vi "Test.vi"() -> ()   [LabVIEW 2014]
uses:
  support/kinectRead [BodyFrame].vi
  <vilib>/vision/NI_Vision_Development_Module.lvlib
panel:
  out "Image":T1(plugin-control)
  in  "stop":bool
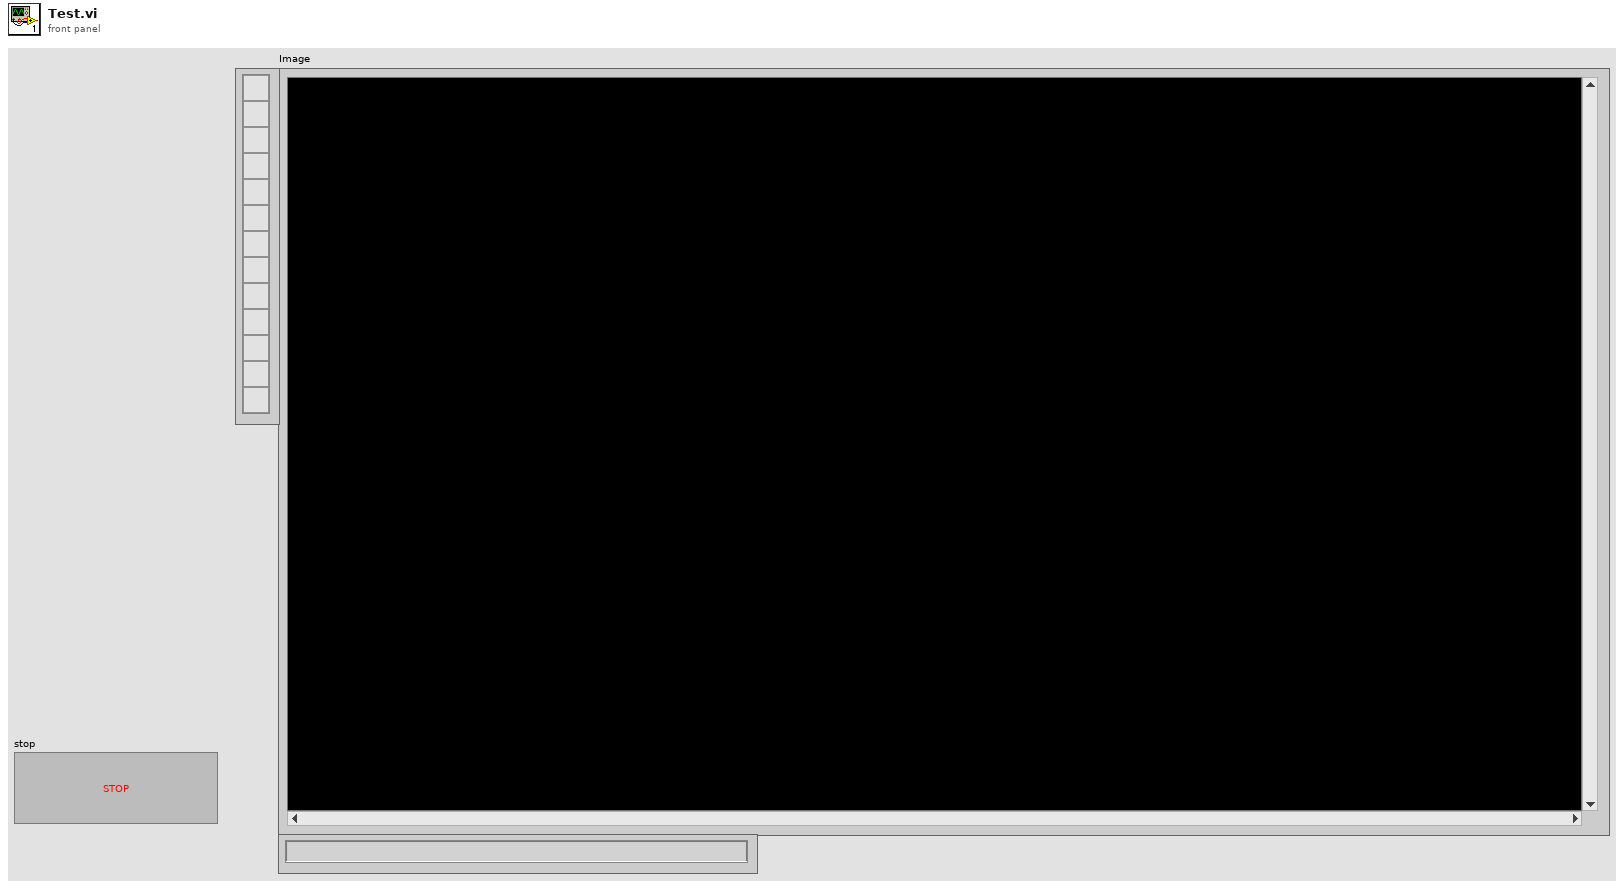
[diagram p1: front panel]
types:
  T1 = typedef "IMAQ Image.ctl" = refnum<image>
  T2 = typedef "Image Type" = u32
  T3 = typedef "KinectSensor References.ctl" = cluster{"KinectSensor":refnum<k24>, "MultiSourceFrameReader":refnum<k24>, "BodyFrameDataInterface":refnum<k24>}
  T4 = typedef "BodyData.ctl" = cluster{"ClippedEdges":i32, "HandLeftConfidence":i32, "HandLeftState":i32, "HandRightConfidence":i32, "HandRightState":i32, "IsRestricted":bool, "IsTracked":bool, "JointOrientations":refnum<k24>, "Joints":refnum<k24>, "Lean":refnum<k24>, "LeanTrackingState":i32, "TrackingId":u64}
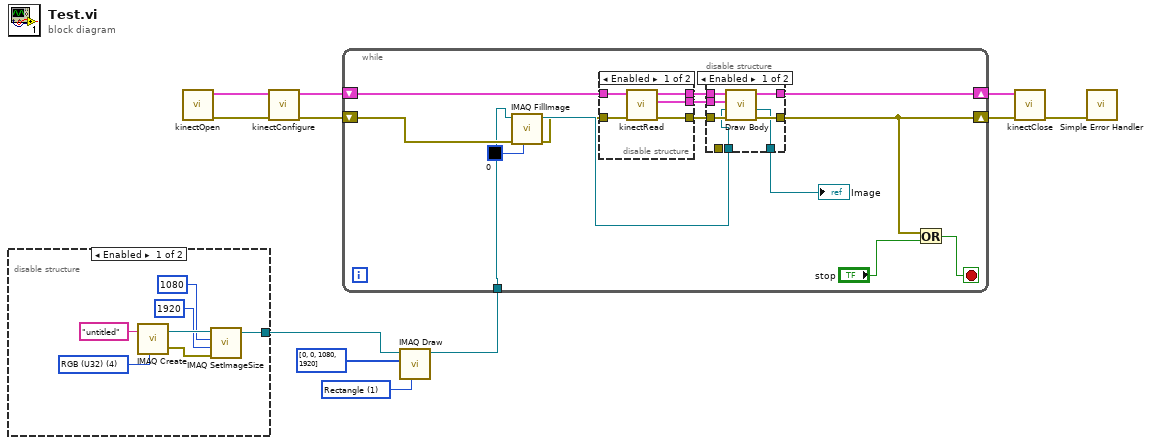
[diagram p0: block diagram]
diagram:
  w4 = u16 1 items=["Line", "Rectangle", "Oval"] ("Shape to draw")
  n1 = disable-structure shown="Enabled" {
    disable-tunnel: [w14 _] -> w2
    frame Enabled {
      w12 = T2 4 items=["Grayscale (U8)", "Grayscale (I16)", "Grayscale (SGL)", "Complex (CSG)", "RGB (U32)", "HSL (U32)", "RGB (U64)", "Grayscale (U16)"] ("Image Type")
      n2 = call "IMAQ Create"("Image Name"="untitled", "Image Type"=w12) -> ("New Image"=w18:T1, "error out"=w17:errorcluster)  [unwired: 3 in]
      n3 = call "IMAQ SetImageSize"("error in (no error)"=w17, "Y Resolution"=1920, "X Resolution"=1080, "Image"=w18) -> ("Image Out"=w14:T1)  [unwired: 1 in, 1 out]
    }
    frame Disabled {
    }
  }
  n4 = call "kinectOpen.vi"() -> ("error out"=w11:errorcluster, "KinectSensor References"=w10:T3)  [unwired: 10 in]
  n5 = call "kinectConfigure.vi"("error in (no error)"=w11, "KinectSensor References in"=w10) -> ("error out"=w5:errorcluster, "KinectSensor References out"=w9:T3)  [unwired: 8 in]
  n6 = call "IMAQ Draw"("Shape to draw"=w4, "Coordinates"=i32[] [0, 0, 1080, 1920], "Image Src"=w2) -> ("Image Dst Out"=w1:T1)  [unwired: 7 in, 1 out]
  n7 = while {
    shift-right: [w29] -> w7
    shift-left: w5 -> [w23]
    shift-right: [w30] -> w8
    shift-left: w9 -> [w24]
    tunnel: w1 -> [w22]
    stop <- w31 stop-if-true
    n8 = call "IMAQ FillImage"("Color Pixel Value"=u32 0, "error in (no error)"=w23, "Image"=w22) -> ("error out"=w19:errorcluster, "Image Out"=w20:T1)  [unwired: 7 in]
    n9 = disable-structure shown="Enabled" {
      disable-tunnel: w24 -> [w37 w39]
      disable-tunnel: [w36 w39] -> w28
      disable-tunnel: [w35 w38] -> w27
      disable-tunnel: [w34 _] -> w26
      disable-tunnel: w19 -> [w33 w38]
      frame Enabled {
        n10 = call-poly "kinectRead.vi"("error in (no error)"=w33, "KinectSensor References in"=w37) -> ("error out"=w35:errorcluster, "Body Data"=w34:T4[], "KinectSensor References out"=w36:T3)  [unwired: 7 in]
      }
      frame Disabled {
      }
    }
    n11 = disable-structure shown="Enabled" {
      disable-tunnel: [w46 w49] -> w30
      disable-tunnel: [w45 w48] -> w29
      disable-tunnel: w28 -> [w44 w49]
      disable-tunnel: w27 -> [w43 w48]
      disable-tunnel: w26 -> [w42 _]
      disable-tunnel: [w41 w47] -> w25
      disable-tunnel: _ -> [_ w47]
      disable-tunnel: w20 -> [w40 _]
      frame Enabled {
        n12 = call "Draw Body.vi"("error in"=w43, "Image"=w40, "Body Data"=w42, "KinectSensor References"=w44) -> ("error out"=w45:errorcluster, "Image Out"=w41:T1, "KinectSensor References out"=w46:T3)  [unwired: 5 in]
      }
      frame Disabled {
      }
    }
    "Image" <- w25
    n13 = Or(x=w29, y="stop") -> (x .or. y?=w31:bool)
  }
  n14 = call "kinectClose.vi"("error in"=w7, "KinectSensor References"=w8) -> ("error out"=w6:errorcluster)  [unwired: 9 in]
  n15 = call <vilib>:"Simple Error Handler.vi"("error in (no error)"=w6) -> ()  [unwired: 4 in, 5 out]
